vi "refresh user interface.vi"(8 "channel names":string[](array[string]), 9 "combo box references":refnum<vi>[](array[refnum]), 10 "engine configuration":refnum<class "engine configuration.lvclass">, 11 "control module configuration in":refnum<class "control module configuration.lvclass">) -> ()   [LabVIEW 2013, in "My Awesome Control Modules editor node.lvclass"]
uses:
  My Awesome Control Modules editor node.lvclass
  <vilib>/NI/Tag Bus Data Framework/control module/configuration/control module configuration.lvclass
  <vilib>/NI/Tag Bus/tag/tag descriptor.lvclass
  <vilib>/NI/Module Execution Interface/Engine Configuration/engine configuration.lvclass
  <vilib>/NI/Configuration Framework/serializable configuration/NISE_CEF_serializable configuration.lvclass
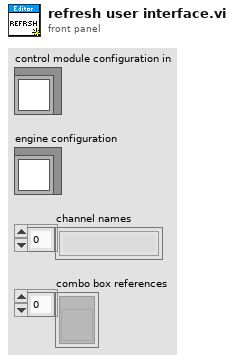
[diagram p1: front panel]
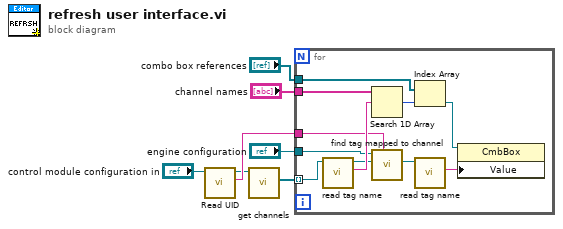
[diagram p0: block diagram]
diagram:
  n1 = call <vilib>:"Read UID.vi"("configuration in"="control module configuration in") -> ("instance id"=w7:string, "configuration out"=w6:refnum<class "control module configuration.lvclass">)  [unwired: 8 in, 1 out]
  n2 = call-dynamic "get channels.vi"("fixed channel configuration in"=w6) -> ("channels"=w2:refnum<class "TBM channel.lvclass">[])  [unwired: 9 in, 1 out]
  n3 = for {
    tunnel: w2 -> [w18] mode=indexing
    tunnel: "channel names" -> [w17]
    tunnel: "combo box references" -> [w14]
    tunnel: "engine configuration" -> [w13]
    tunnel: w7 -> [w12]
    n4 = call <vilib>:"read tag name.vi"("system tag in"=w18) -> ("name"=w16:string, "system tag out"=w11:refnum<class "TBM channel.lvclass">)  [unwired: 8 in, 1 out]
    n5 = Search 1D Array(1D array=w17, element=w16) -> (index of element=w15:i32)  [unwired: 1 in]
    n6 = call <vilib>:"find tag mapped to channel.vi"("owner"=w12, "channel"=w11, "engine configuration in"=w13) -> ("tag"=w10:refnum<class "tag descriptor.lvclass">)  [unwired: 6 in, 2 out]
    n7 = Index Array(array=w14, index=w15) -> (element=w9:refnum<vi>)
    n8 = call <vilib>:"read tag name.vi"("system tag in"=w10) -> ("name"=w8:string)  [unwired: 8 in, 2 out]
    n9 = property class="CmbBox"(reference=w9, "Value"=w8) -> ()  [unwired: 1 in, 2 out]
  }
